vi "Abort.vi"() -> ()   [LabVIEW 2015]
panel:
  in  "Abort":bool
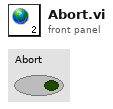
[diagram p1: front panel]
diagram:
